vi "SPI API - SPI Simulation.vi"() -> ()   [LabVIEW 2014]
uses:
  Controls/Timing Characteristics.ctl
  Controls/Digital Data.ctl
  <vilib>/rvi/DesktopExecutionNode/Execution/niFpgaDEN_Execute.vi
  <vilib>/rvi/DesktopExecutionNode/DesktopExecutionNode.xnode
panel:
  out "Data To Slave":u64 format="%b"
  out "Timing Characteristics":T1 {"tCL (ns)" format="%#_4g"; "tCH (ns)" format="%#_4g"; "tCP (ns)" format="%#_4g"; "tCSS (ns)" format="%#_4g"; "tCSH (ns)" format="%#_4g"; "tCSW (ns)" format="%#_4g"; "Actual Sample Rate (Hz)" format="%_4p"; "SCLK Frequency (Hz)" format="%#.2p"}
  in  "Pause":bool
  in  "SPI PHY Settings":T2={"Divide Value"=10, "Transfer Length (bits)"=24, "CS Asserted Polarity"=FALSE, "Clock Polarity (CPOL)"=FALSE, "Clock Phase (CPHA)"=FALSE, "Lengthen MISO Setup"=FALSE, "Direction Change Bit"=0, "MOSI Starts as Output"=FALSE, "Tristatable MOSI"=FALSE}
  in  "Sample Rate (Hz)":u32=75000
  out "Digital Data":digitalwaveform(graph)
  in  "Data To Slave":u64
  in  "Stop":bool
  # "Operating Instructions\n1. For this VI to work, the FPGA must be in Simulation Mode.\n2. Run the VI and change the 'SPI PHY Settings' and 'Data To Slave' controls to change the SPI Output.\n3. While changing the settings, view the timing characteristics of the signal on the right side of the graph."
  # "Typical Timing Diagram"
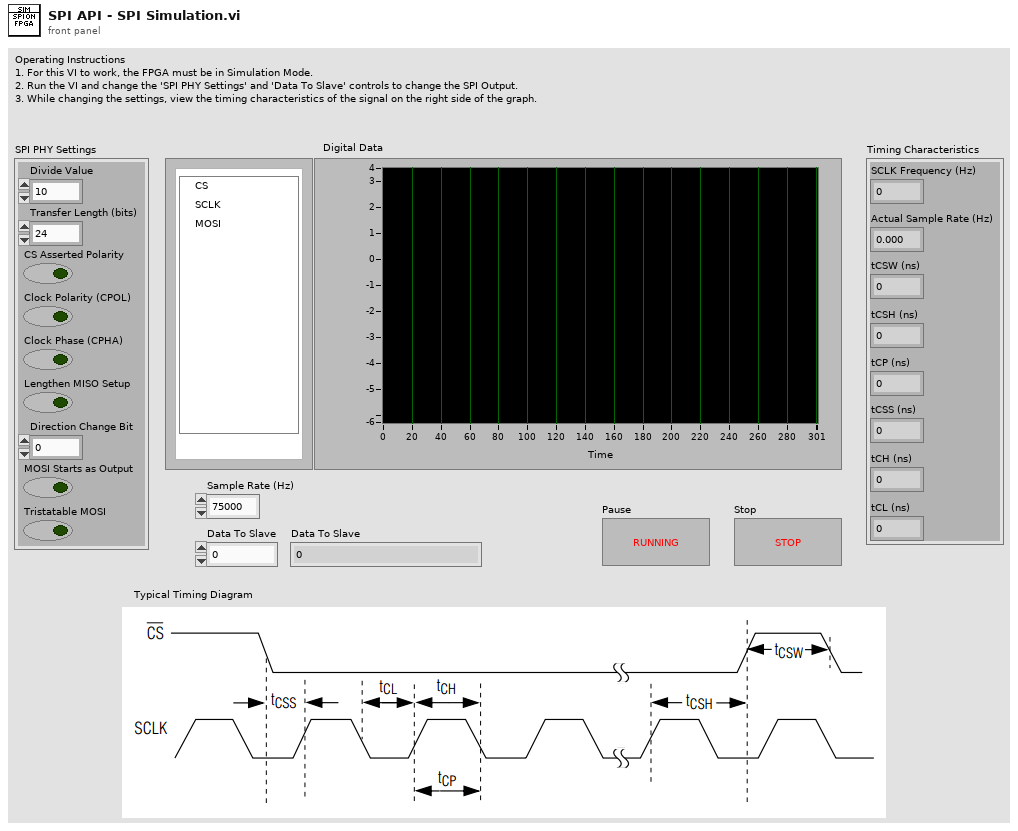
[diagram p1: front panel]
types:
  T1 = typedef "Timing Characteristics.ctl" = cluster{"SCLK Frequency (Hz)":dbl, "Actual Sample Rate (Hz)":dbl, "tCSW (ns)":dbl, "tCSH (ns)":dbl, "tCSS (ns)":dbl, "tCP (ns)":dbl, "tCH (ns)":dbl, "tCL (ns)":dbl}
  T2 = cluster{"Divide Value":u8, "Transfer Length (bits)":u8, "CS Asserted Polarity":bool, "Clock Polarity (CPOL)":bool, "Clock Phase (CPHA)":bool, "Lengthen MISO Setup":bool, "Direction Change Bit":u8, "MOSI Starts as Output":bool, "Tristatable MOSI":bool}
  T3 = typedef "Digital Data.ctl" = cluster{"CS":bool, "SCLK":bool, "MISO":bool}
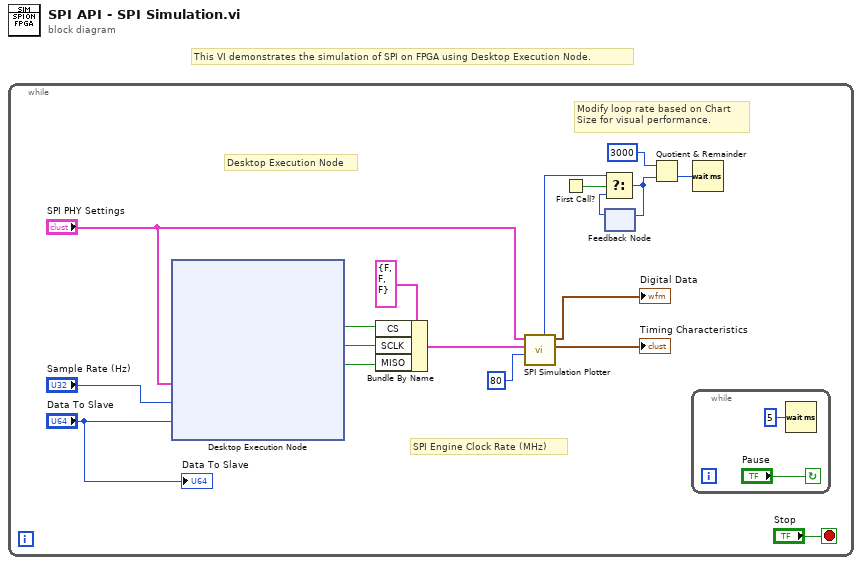
[diagram p0: block diagram]
diagram:
  # "This VI demonstrates the simulation of SPI on FPGA using Desktop Execution Node."
  n1 = while {
    stop <- "Stop" stop-if-true
    # "Desktop Execution Node"
    # "SPI Engine Clock Rate (MHz)"
    # "Modify loop rate based on Chart\nSize for visual performance."
    n2 = xnode "Desktop Execution Node"("SPI PHY Settings"="SPI PHY Settings", "Data Rate (S/s)"="Sample Rate (Hz)", "Data To Slave"="Data To Slave") -> ("CS"=w6:bool, "SCLK"=w5:bool, "MOSI"=w4:bool)  [unwired: 1 in, 1 out]
    n3 = Bundle By Name(cluster=T3 {"CS"=FALSE, "SCLK"=FALSE, "MISO"=FALSE}, "CS"=w6, "SCLK"=w5, "MISO"=w4) -> (w11:T3)
    n4 = call "SPI Simulation Plotter.vi"("Engine Clock Rate (MHz)"=80, "SPI Signals"=w11, "SPI PHY Settings"="SPI PHY Settings") -> ("Timing Characteristics"=→"Timing Characteristics":T1, "Digital Data"=→"Digital Data":digitalwaveform, "Chart Size"=w10:i32)  [unwired: 6 in]
    n5 = First Call?() -> (First Call?: T/F=w16:bool)
    n6 = feedback #1() -> (w15:i32)  [unwired: 1 in]
    n7 = Select(t=w10, s=w16, f=w15) -> (s? t:f=w14:i32)
    n8 = feedback-in #1(w14) -> ()
    n9 = Quotient & Remainder(x=u32 3000 ("ms per Command"), y=w14) -> (floor(x/y)=w12:u32)  [unwired: 1 out]
    n10 = while {
      stop <- "Pause" continue-if-true
      n11 = Wait (ms)(milliseconds to wait=u32 5) -> ()  [unwired: 1 out]
    }
    n12 = Wait (ms)(milliseconds to wait=w12) -> ()  [unwired: 1 out]
    "Data To Slave" <- "Data To Slave"
  }
